vi "Divide Output Gain.vi"(8 "error in (no error)":errorcluster, 10 "WFM in":waveform(dbl)[](array[waveform]), 11 "Instrument.DAQ":refnum<class "Instrument.DAQ.lvclass">) -> (0 "error out":errorcluster, 2 "WFM out":waveform(dbl)[](array[waveform]), 3 "Instrument.DAQ out":refnum<class "Instrument.DAQ.lvclass">)   [LabVIEW 2019, in "Instrument.DAQ.lvclass"]
uses:
  Instrument.DAQ.lvclass
  Instrument.DAQ.lvclass/Instrument.DAQ.ctl
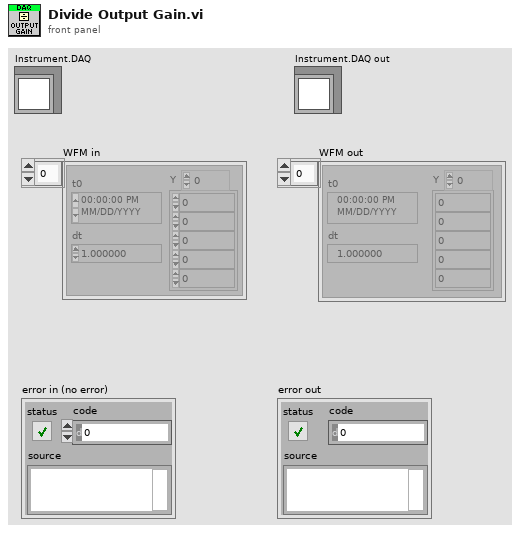
[diagram p1: front panel]
types:
  T1 = typedef "Instrument.DAQ.lvclass/Channel.Gain--Cluster--Array.ctl" = T2[]
  T2 = typedef "Instrument.DAQ.lvclass/Channel.Gain--Cluster.ctl" = cluster{"Channel":string, "Gain":dbl}
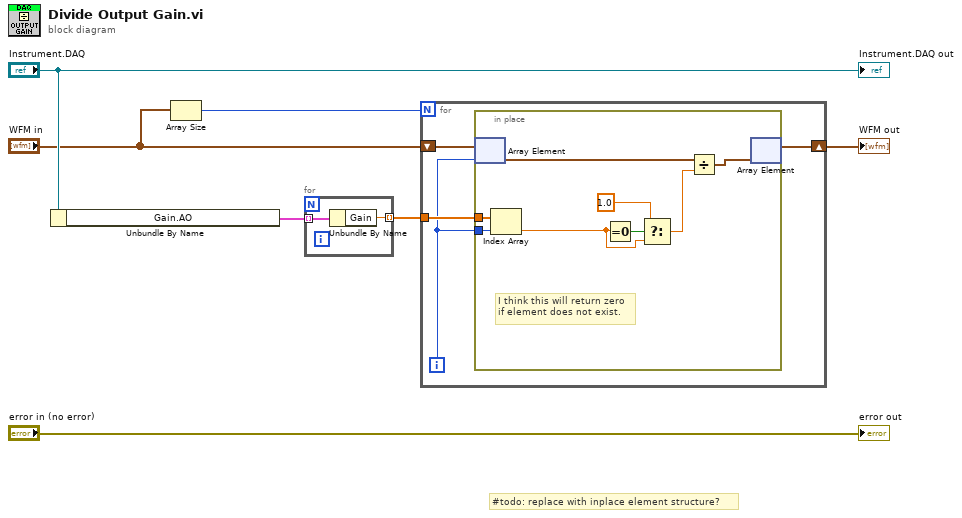
[diagram p0: block diagram]
diagram:
  # "#todo: replace with inplace element structure?"
  n1 = Unbundle By Name("Instrument.DAQ") -> ("Gain.AO"=w2:T1)
  n2 = Array Size(array="WFM in") -> (size(s)=w3:i32)
  n3 = for {
    tunnel: w2 -> [w9] mode=indexing
    tunnel: [w8] -> w1 mode=indexing
    n4 = Unbundle By Name(w9) -> ("Gain"=w8:dbl)
  }
  n5 = for {
    N: w3 -> [_]
    tunnel: w1 -> [w13]
    shift-right: [w12] -> w7
    shift-left: "WFM in" -> [w10]
    i -> [w11]
    n6 = in-place {
      in-place-border: w11 -> [w21]
      in-place-border: w13 -> [w20]
      # "I think this will return zero\nif element does not exist."
      n7 = in-place-array #1(w10, w11) -> (w16:waveform(dbl))
      n8 = Index Array(array=w20, index=w21) -> (element=w14:dbl)
      n9 = Equal To 0?(x=w14) -> (x = 0?=w19:bool)
      n10 = Select(t=1.0, s=w19, f=w14) -> (s? t:f=w18:dbl)
      n11 = Divide(x=w16, y=w18) -> (x/y=w15:waveform(dbl))
      n12 = in-place-array #1(w15) -> (w12:waveform(dbl)[])  [unwired: 1 out]
    }
  }
  "WFM out" <- w7
  "error out" <- "error in (no error)"
  "Instrument.DAQ out" <- "Instrument.DAQ"
